vi "PH_gentec_Powermeter.PC Start Stop Statistics.vi"(0 "VI in":refnum<vi>, 2 "Start / Stop Statistics":bool, 5 "error in (no error)":errorcluster) -> (14 "VI out":refnum<vi>, 19 "error out":errorcluster)   [LabVIEW 2014, in "PH_gentec_Powermeter.lvlib"]
uses:
  PH_gentec_Powermeter.lvlib
  PH_Common/PH_Common.lvlib
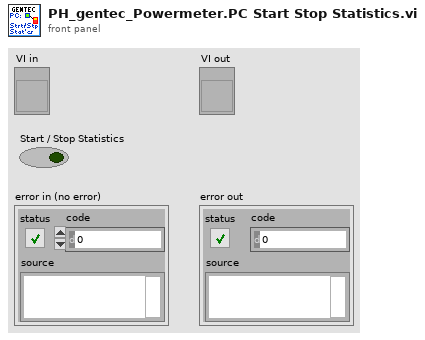
[diagram p1: front panel]
types:
  T1 = typedef "PH_gentec_Powermeter.lvlib/PH_gentec_Powermeter.i attribute.ctl" = cluster{"GUI References":cluster{"delete":refnum<vi>, "start stop Statistics":refnum<vi>, "Statistic Data":refnum<vi>, "Configuration Values":refnum<vi>, "Set Zero":refnum<vi>, "Data Sampling Settings":refnum<vi>, "Wanted Sets":refnum<vi>, "Current Sets":refnum<vi>}, "Start Stop Statistics":bool, "Wanted Sets":T2, "Current Sets":T2}
  T2 = typedef "PH_gentec_Powermeter.lvlib/PH_gentec_Powermeter.Sets.ctl" = cluster{"Data Sampling Settings":T3, "Set Zero":bool}
  T3 = typedef "gentec-SOLO-PE - Driver.lvlib/gentec-SOLO-PE.Data Sampling Settings.ctl" = cluster{"Sample Rate":u32, "Sample Rate Unit":u32, "Sample Period":u32, "Sample Period Unit":u32, "Total Duration":u32, "Total Duration Unit":u32, "Time Stamp":u32}
  T4 = enum8{"Enabled", "Disabled", "Disabled and Grayed Out"}
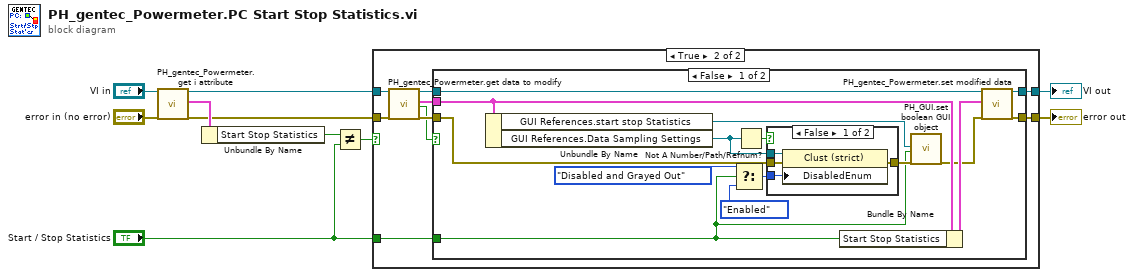
[diagram p0: block diagram]
diagram:
  n1 = call "PH_gentec_Powermeter.get i attribute.vi"("i ref in"="VI in", "error in (no error)"="error in (no error)") -> ("i ref out"=w6:refnum<vi>, "i attribute"=w7:T1, "error out"=w4:errorcluster)  [unwired: 15 in]
  n2 = Unbundle By Name(w7) -> ("Start Stop Statistics"=w8:bool)
  n3 = Not Equal?(x=w8, y="Start / Stop Statistics") -> (x != y?=w10:bool)
  n4 = case shown="True" w10 {
    tunnel: [w11 w20] -> w2
    tunnel: [w12 w18] -> w3
    tunnel: w4 -> [w11 w15]
    tunnel: w6 -> [w12 w14]
    tunnel: "Start / Stop Statistics" -> [_ w13]
    frame False {
    }
    frame True {
      n5 = call "PH_gentec_Powermeter.get data to modify.vi"("i ref in"=w14, "error in (no error)"=w15) -> ("i ref out"=w19:refnum<vi>, "i attribute"=w17:T1, "timed out"=w16:bool, "error out"=w21:errorcluster)  [unwired: 14 in]
      n6 = case shown="False" w16 {
        tunnel: w21 -> [w36 w42]
        tunnel: [w29 w42] -> w20
        tunnel: w19 -> [w35 w43]
        tunnel: [w30 w43] -> w18
        tunnel: w17 -> [w33 _]
        tunnel: w13 -> [w27 _]
        frame False {
          n7 = Unbundle By Name(w33) -> ("GUI References.start stop Statistics"=w31:refnum<vi>, "GUI References.Data Sampling Settings"=w24:refnum<vi>)
          n8 = Select(t=T4."Disabled and Grayed Out" ("Disabled"), s=w27, f=T4."Enabled" ("Disabled")) -> (s? t:f=w26:T4)
          n9 = Not A Number/Path/Refnum?(number/path/refnum=w24) -> (NaN/Path/Refnum?=w25:bool)
          n10 = case shown="False" w25 {
            tunnel: w36 -> [w40 w41]
            tunnel: [w39 w41] -> w28
            tunnel: w24 -> [w38 _]
            tunnel: w26 -> [w37 _]
            frame False {
              n11 = property class="Clust (strict)"(reference=w38, error in=w40, "DisabledEnum"=w37) -> (error out=w39:errorcluster)  [unwired: 1 out]
            }
            frame True {
            }
          }
          n12 = Bundle By Name(cluster=w33, "Start Stop Statistics"=w27) -> (w34:T1)
          n13 = call "PH_GUI.set boolean GUI object.vi"("Boolean Knob GUI Ref"=w31, "Value"=w27, "error in (no error)"=w28) -> ("error out"=w32:errorcluster)  [unwired: 16 in]
          n14 = call "PH_gentec_Powermeter.set modified data.vi"("i ref in"=w35, "i attribute"=w34, "error in (no error)"=w32) -> ("i ref out"=w30:refnum<vi>, "error out"=w29:errorcluster)  [unwired: 15 in]
        }
        frame True {
        }
      }
    }
  }
  "VI out" <- w3
  "error out" <- w2
